vi "SGL to Hex.vi"(11 "Data":sgl) -> (3 "HexData":string)   [LabVIEW 2017]
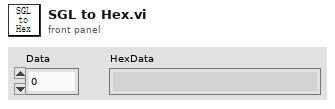
[diagram p1: front panel]
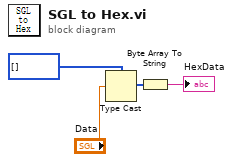
[diagram p0: block diagram]
diagram:
  n1 = Type Cast(type=u8[] [], x="Data") -> (*(type *) &x=w2:u8[])
  n2 = Byte Array To String(unsigned byte array=w2) -> (string=→"HexData":string)
